vi "as INT32.vi"(11 "bytes":u8[](array[numeric]) format="%b") -> (3 "INT32":i32)   [LabVIEW 2020, in "MessagePack.lvlib" / "MessagePackNumeric.lvclass"]
uses:
  MessagePackNumeric.lvclass
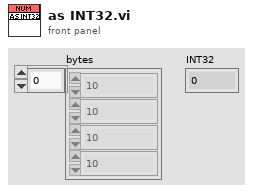
[diagram p1: front panel]
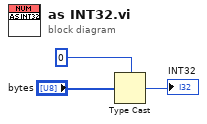
[diagram p0: block diagram]
diagram:
  n1 = Type Cast(type=0 ("INT8"), x="bytes") -> (*(type *) &x=→"INT32":i32)
